vi "temporalTowOdorsDiscrimnation.vi"() -> ()   [LabVIEW 2011]
uses:
  <vilib>/Utility/file.llb/Write To Spreadsheet File (DBL).vi
  <vilib>/DAQmx/write.llb/DAQmx Write (Analog DBL 1Chan 1Samp).vi
  <vilib>/DAQmx/create/channels.llb/DAQmx Create Channel (DO-Digital Output).vi
panel:
  out "loop 2":i32
  out "loop 1":i32
  out "Only B flag":dbl
  out "Only A  flag":dbl
  out "Stop on":bool
  out "file open":bool=TRUE
  in  "Save file":bool
  in  "base path":path=path "C:/Code/Matan/Lower Setup/1.6.14/Mouse 1"
  in  "name":string="6.1.14_Mouse 1"
  out "appended path":path=path "C:/Code/Matan/Lower Setup/1.6.14/Mouse 1/6.1.14_Mouse 1_010614132538.DAT"
  in  "?":T1(radio)
  out "#Correct":dbl
  out "Success rate":dbl(knob) scale=0.0..100.0
  out "B port value":dbl
  out "A port value":dbl
  out "Selected odor number":dbl
  in  "Delta T":dbl
  out "Odor identity?":bool
  in  "ISI":dbl
  out "Trial #":dbl
  out "User instructions":string
  in  "Trials number":i32
  out "Prot value":dbl
  in  "Odor duration":dbl
  out "Odor B start time":dbl
  out "Odor A start time":dbl
  # "Results"
  # "Calculated parameters"
  # "Parameters"
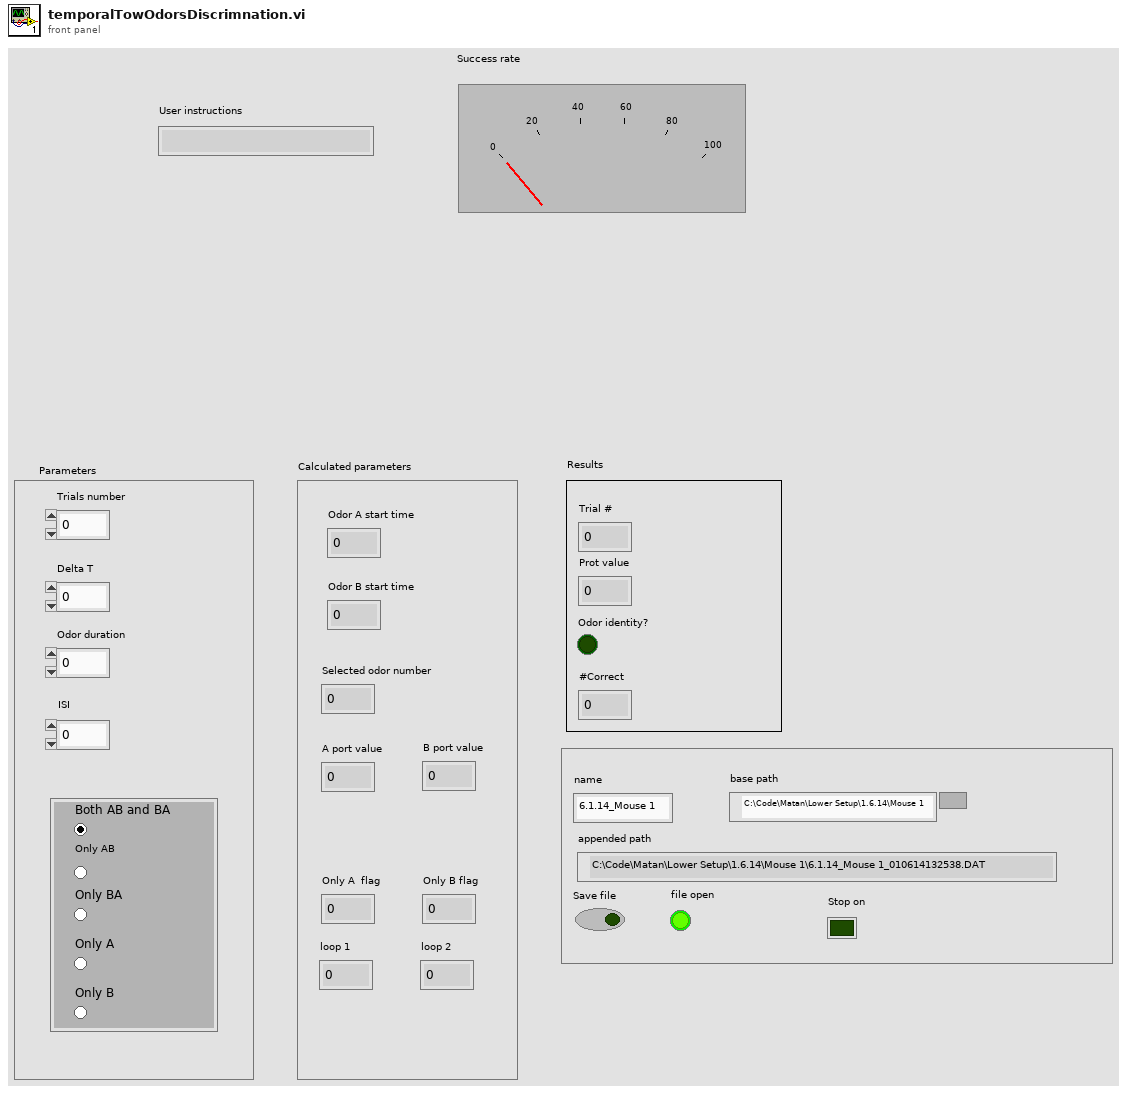
[diagram p1: front panel]
types:
  T1 = enum32{"Both AB and BA", "Only AB", "Only BA", "Only A", "Only B"}
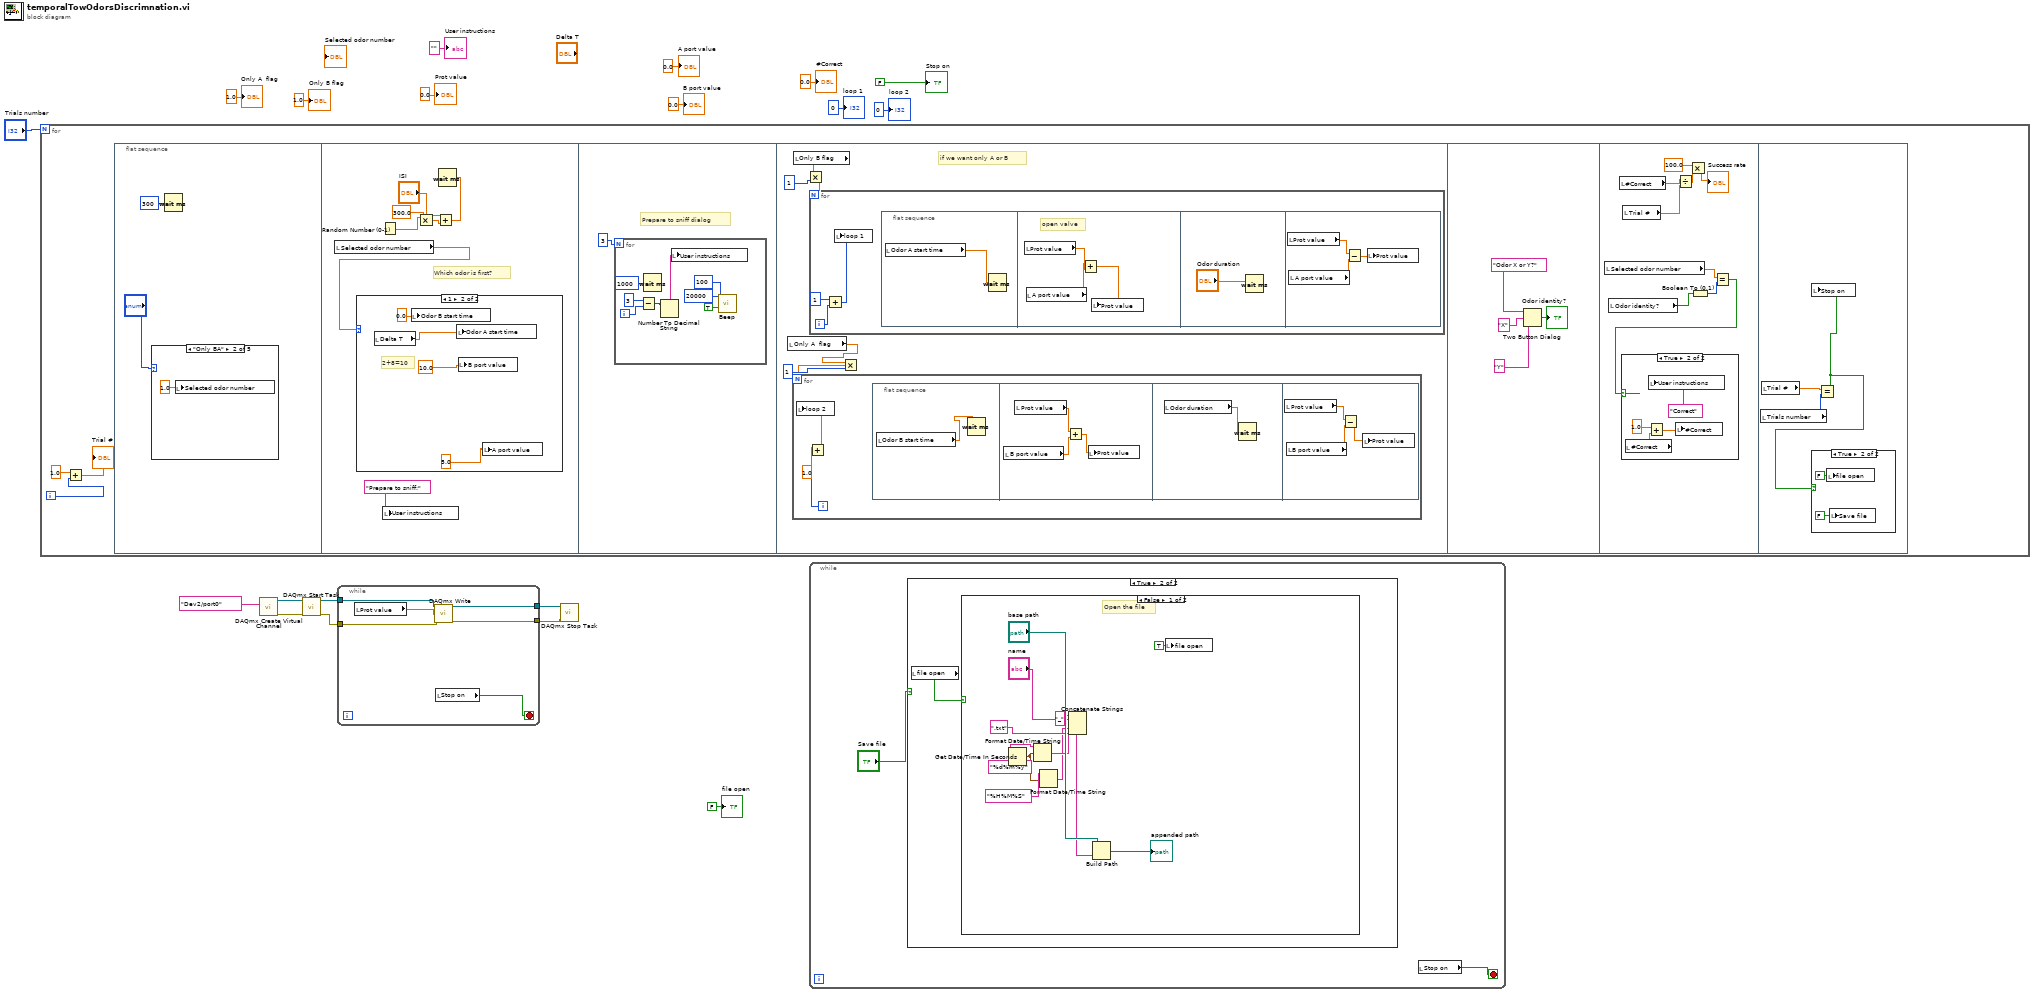
[diagram p0: block diagram]
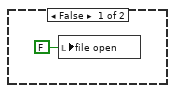
[diagram p2: hidden frame]
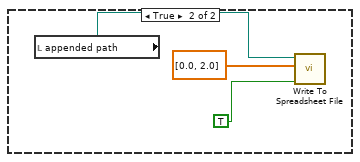
[diagram p3: hidden frame]
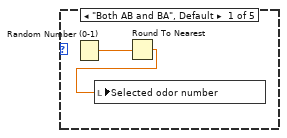
[diagram p4: hidden frame]
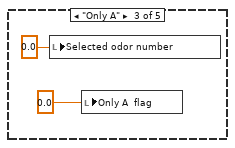
[diagram p5: hidden frame]
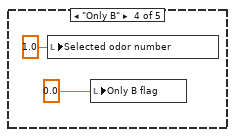
[diagram p6: hidden frame]
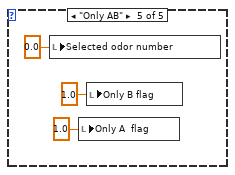
[diagram p7: hidden frame]
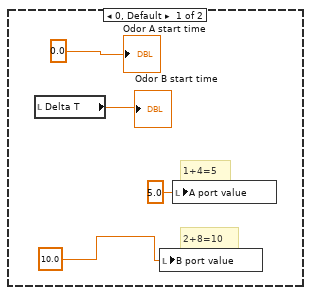
[diagram p8: hidden frame]
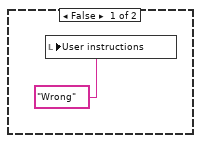
[diagram p9: hidden frame]
diagram:
  n1 = for {
    N: "Trials number" -> [_]
    i -> [w21]
    n2 = Add(x=1.0, y=w21) -> (x+y=→"Trial #":dbl)
    n3 = flat-sequence {
      frame #0 {
        n4 = case shown="\"Only BA\"" "?" {
          frame "Both AB and BA", Default {
            n5 = Random Number (0-1)() -> (number: 0 to 1=w26:dbl)
            n6 = Round To Nearest(number=w26) -> (nearest integer value=w25:dbl)
            n7 = local write "Selected odor number"(w25) -> ()
          }
          frame "Only BA" {
            n8 = local write "Selected odor number"(1.0 ("Selected odor number")) -> ()
          }
          frame "Only A" {
            n9 = local write "Selected odor number"(0.0 ("Selected odor number")) -> ()
            n10 = local write "Only A  flag"(0.0 ("A or  B alone flag")) -> ()
          }
          frame "Only B" {
            n11 = local write "Selected odor number"(1.0 ("Selected odor number")) -> ()
            n12 = local write "Only B flag"(0.0 ("A or  B alone flag")) -> ()
          }
          frame "Only AB" {
            n13 = local write "Selected odor number"(0.0 ("Selected odor number")) -> ()
            n14 = local write "Only A  flag"(1.0 ("Only A  flag")) -> ()
            n15 = local write "Only B flag"(1.0 ("Only B flag")) -> ()
          }
        }
        n16 = Wait (ms)(milliseconds to wait=u32 300) -> ()  [unwired: 1 out]
      }
      frame #1 {
        # "Which odor is first?"
        n17 = local read "Selected odor number"() -> (w35:dbl)
        n18 = case shown="1" w35 {
          frame 0, Default {
            # "2+8=10"
            # "1+4=5"
            n19 = local read "Delta T"() -> (→"Odor B start time":dbl)
            n20 = local write "B port value"(10.0 ("B port value")) -> ()
            n21 = local write "A port value"(5.0 ("A port value")) -> ()
            "Odor A start time" <- 0.0 ("Odor A start time")
          }
          frame 1 {
            # "2+8=10"
            n22 = local read "Delta T"() -> (w49:dbl)
            n23 = local write "Odor B start time"(0.0 ("Odor B start time")) -> ()
            n24 = local write "Odor A start time"(w49) -> ()
            n25 = local write "B port value"(10.0 ("A port value")) -> ()
            n26 = local write "A port value"(5.0 ("B port value")) -> ()
          }
        }
        n27 = Random Number (0-1)() -> (number: 0 to 1=w37:dbl)
        n28 = local write "User instructions"("Prepare to sniff:" ("User instructions")) -> ()
        n29 = Multiply(x=w37, y=300.0) -> (x*y=w39:dbl)
        n30 = Add(x="ISI", y=w39) -> (x+y=w41:dbl)
        n31 = Wait (ms)(milliseconds to wait=w41) -> ()  [unwired: 1 out]
      }
      frame #2 {
        # "Prepare to sniff dialog"
        n32 = for {
          N: 3 -> [_]
          i -> [w56]
          n33 = Subtract(x=3, y=w56) -> (x-y=w55:i32)
          n34 = Wait (ms)(milliseconds to wait=u32 1000) -> ()  [unwired: 1 out]
          n35 = Number To Decimal String(number=w55) -> (decimal integer string=w57:string)  [unwired: 1 in]
          n36 = local write "User instructions"(w57) -> ()
          n37 = call <vilib>:"Beep.vi"("use system alert? (T)"=TRUE, "duration (msec)"=u32 100, "frequency (Hz)"=u32 20000) -> ()  [unwired: 9 in]
        }
      }
      frame #3 {
        # "if we want only A or B"
        n38 = local read "Only A  flag"() -> (w60:dbl)
        n39 = local read "Only B flag"() -> (w59:dbl)
        n40 = Multiply(x=w59, y=1) -> (x*y=w64:dbl)
        n41 = for {
          N: w64 -> [_]
          i -> [w78]
          n42 = Add(x=1, y=w78) -> (x+y=w76:i32)
          n43 = local write "loop 1"(w76) -> ()
          n44 = flat-sequence {
            frame #0 {
              n45 = local read "Odor A start time"() -> (w79:dbl)
              n46 = Wait (ms)(milliseconds to wait=w79) -> ()  [unwired: 1 out]
            }
            frame #1 {
              # "open valve"
              n47 = local read "Prot value"() -> (w82:dbl)
              n48 = local read "A port value"() -> (w81:dbl)
              n49 = Add(x=w81, y=w82) -> (x+y=w80:dbl)
              n50 = local write "Prot value"(w80) -> ()
            }
            frame #2 {
              n51 = Wait (ms)(milliseconds to wait="Odor duration") -> ()  [unwired: 1 out]
            }
            frame #3 {
              n52 = local read "Prot value"() -> (w86:dbl)
              n53 = local read "A port value"() -> (w84:dbl)
              n54 = Subtract(x=w86, y=w84) -> (x-y=w85:dbl)
              n55 = local write "Prot value"(w85) -> ()
            }
          }
        }
        n56 = Multiply(x=w60, y=1) -> (x*y=w61:dbl)
        n57 = for {
          N: w61 -> [_]
          i -> [w66]
          n58 = Add(x=1.0, y=w66) -> (x+y=w65:dbl)
          n59 = local write "loop 2"(w65) -> ()
          n60 = flat-sequence {
            frame #0 {
              n61 = local read "Odor B start time"() -> (w68:dbl)
              n62 = Wait (ms)(milliseconds to wait=w68) -> ()  [unwired: 1 out]
            }
            frame #1 {
              n63 = local read "B port value"() -> (w69:dbl)
              n64 = local read "Prot value"() -> (w71:dbl)
              n65 = Add(x=w71, y=w69) -> (x+y=w70:dbl)
              n66 = local write "Prot value"(w70) -> ()
            }
            frame #2 {
              n67 = local read "Odor duration"() -> (w72:dbl)
              n68 = Wait (ms)(milliseconds to wait=w72) -> ()  [unwired: 1 out]
            }
            frame #3 {
              n69 = local read "Prot value"() -> (w74:dbl)
              n70 = local read "B port value"() -> (w73:dbl)
              n71 = Subtract(x=w74, y=w73) -> (x-y=w75:dbl)
              n72 = local write "Prot value"(w75) -> ()
            }
          }
        }
      }
      frame #4 {
        n73 = Two Button Dialog(message="Odor X or Y?", 1:"Y" ("F button name (\"Cancel\")"), 2:"X" ("T button name (\"OK\")")) -> (T button?=→"Odor identity?":bool)
      }
      frame #5 {
        n74 = local read "Selected odor number"() -> (w97:dbl)
        n75 = local read "Odor identity?"() -> (w99:bool)
        n76 = local read "#Correct"() -> (w95:dbl)
        n77 = local read "Trial #"() -> (w91:dbl)
        n78 = Divide(x=w95, y=w91) -> (x/y=w93:dbl)
        n79 = Multiply(x=100.0, y=w93) -> (x*y=→"Success rate":dbl)
        n80 = Boolean To (0,1)(Boolean=w99) -> (0, 1=w98:i16)
        n81 = Equal?(x=w97, y=w98) -> (x = y?=w96:bool)
        n82 = case shown="True" w96 {
          frame False {
            n83 = local write "User instructions"("Wrong" ("User instructions")) -> ()
          }
          frame True {
            n84 = local read "#Correct"() -> (w101:dbl)
            n85 = Add(x=1.0, y=w101) -> (x+y=w103:dbl)
            n86 = local write "User instructions"("Correct" ("User instructions")) -> ()
            n87 = local write "#Correct"(w103) -> ()
          }
        }
      }
      frame #6 {
        n88 = local read "Trials number"() -> (w107:i32)
        n89 = local read "Trial #"() -> (w106:dbl)
        n90 = Equal?(x=w106, y=w107) -> (x = y?=w105:bool)
        n91 = local write "Stop on"(w105) -> ()
        n92 = case shown="True" w105 {
          frame False {
          }
          frame True {
            n93 = local write "file open"(FALSE ("file open")) -> ()
            n94 = local write "Save file"(FALSE ("Save file")) -> ()
          }
        }
      }
    }
  }
  n95 = call-poly <vilib>:"DAQmx Create Virtual Channel.vi"("lines"=tag "Dev2/port0") -> ("task out"=w13:refnum<k21>, "error out"=w12:errorcluster)  [unwired: 13 in]
  n96 = call <vilib>:"DAQmx Start Task.vi"("task/channels in"=w13, "error in"=w12) -> ("task out"=w10:refnum<k21>, "error out"=w9:errorcluster)  [unwired: 12 in]
  n97 = while {
    tunnel: w10 -> [w115]
    tunnel: [w114] -> w2
    tunnel: [w113] -> w1
    tunnel: w9 -> [w112]
    stop <- w110 stop-if-true
    n98 = local read "Prot value"() -> (w111:dbl)
    n99 = call-poly <vilib>:"DAQmx Write.vi"("task/channels in"=w115, "data"=w111, "error in"=w112) -> ("task out"=w114:refnum<k21>, "error out"=w113:errorcluster)  [unwired: 10 in, 1 out]
    n100 = local read "Stop on"() -> (w110:bool)
  }
  n101 = call <vilib>:"DAQmx Stop Task.vi"("task/channels in"=w2, "error in"=w1) -> ()  [unwired: 12 in, 2 out]
  n102 = while {
    stop <- w116 stop-if-true
    n103 = case shown="True" "Save file" {
      frame False {
        n104 = local write "file open"(FALSE ("file open")) -> ()
      }
      frame True {
        n105 = local read "file open"() -> (w119:bool)
        n106 = case shown="False" w119 {
          frame False {
            # "Open the file"
            n107 = Get Date/Time In Seconds() -> (seconds since 1Jan1904=w126:timestamp)
            n108 = Format Date/Time String(time format string (%c)="%d%m%y", seconds (now)=w126) -> (date/time string=w124:string)  [unwired: 1 in]
            n109 = Format Date/Time String(time format string (%c)="%H%M%S", seconds (now)=w126) -> (date/time string=w123:string)  [unwired: 1 in]
            n110 = Concatenate Strings("name", "_" ("string"), w124, w123, ".txt") -> (w129:string)
            n111 = Build Path(base path="base path", name or relative path=w129) -> (appended path=→"appended path":path)
            n112 = local write "file open"(TRUE ("file open")) -> ()
          }
          frame True {
            n113 = local read "appended path"() -> (w134:path)
            n114 = call-poly <vilib>:"Write To Spreadsheet File.vi"("append to file? (new file:F)"=TRUE, "1D data"=dbl[] [0.0, 2.0], "file path (dialog if empty)"=w134) -> ()  [unwired: 5 in, 1 out]
          }
        }
      }
    }
    n115 = local read "Stop on"() -> (w116:bool)
  }
  "Prot value" <- 0.0 ("Prot value")
  "User instructions" <- "" ("User instructions")
  "A port value" <- 0.0 ("A port value")
  "B port value" <- 0.0 ("B port value")
  "#Correct" <- 0.0 ("#Correct")
  "Stop on" <- FALSE ("Stop on")
  "file open" <- FALSE ("file open")
  "Only A  flag" <- 1.0 ("A or  B alone flag")
  "Only B flag" <- 1.0 ("Only B flag")
  "loop 1" <- 0 ("loop 1")
  "loop 2" <- 0 ("loop 2")
